vi "Teleop.vi"(10 "Match Info":T1={"Autonomous Elapsed Seconds"=0.0, "TeleOp Elapsed Seconds"=0.0, "Disabled Elapsed Seconds"=0.0, "Visited Autonomous"=FALSE, "Visited TeleOp"=FALSE, "Visited Disabled"=FALSE, "Autonomous Settings"={"Autonomous Style"=enum."Independent", "VI Refnum"=refnum}}, 11 "Call Context":T2) -> ()   [LabVIEW 2019]
doc: "This VI is called for each TeleOp packet received from the DS where the robot is not disabled. It is often used to read from the joysticks and update I/O or to update setpoints for timed control loops. It should complete and return within 20 milliseconds or it may miss DS packets."
uses:
  <vilib>/Rock Robotics/Network Tables/NT Read Boolean.vi
  Robot Global Data.vi
  <vilib>/Rock Robotics/WPI/Joystick/WPI_JoystickArcadeMapping.vi
  <vilib>/Rock Robotics/Network Tables/NT Read Number.vi
  <vilib>/Rock Robotics/Network Tables/NT Write Boolean Array.vi
  <vilib>/Rock Robotics/Network Tables/NT Write Numeric Array.vi
  <vilib>/Rock Robotics/WPI/ThirdParty/JAS_Junk/TrajLib/Trajectory_Library.lvlib
  <vilib>/Rock Robotics/WPI/DriverStation/WPI_DriverStationMatch Info.ctl
  <vilib>/Rock Robotics/WPI/DriverStation/WPI_DriverStationDerivedRobotMode.ctl
panel:
  out "Sample Slider 0":dbl(slide) scale=0.0..5.0
  out "Sample Boolean 1":bool
  out "Sample Boolean 0":bool
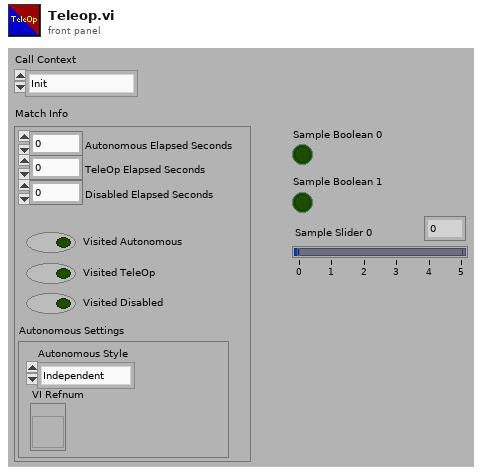
[diagram p1: front panel]
types:
  T1 = typedef "WPI_DriverStationMatch Info.ctl" = cluster{"Autonomous Elapsed Seconds":dbl, "TeleOp Elapsed Seconds":dbl, "Disabled Elapsed Seconds":dbl, "Visited Autonomous":bool, "Visited TeleOp":bool, "Visited Disabled":bool, "Autonomous Settings":cluster{"Autonomous Style":enum16{"Iterative", "Independent"}, "VI Refnum":refnum<vi>}}
  T2 = typedef "WPI_DriverStationDerivedRobotMode.ctl" = enum16{"Init", "Execute", "Stop"}
  T3 = typedef "WPI_JoystickDevRef.ctl" = cluster{"Device":T4}
  T4 = typedef "WPI_JoystickDeviceEnum.ctl" = enum16{"USB 0", "USB 1", "USB 2", "USB 3", "USB 4", "USB 5"}
  T5 = typedef "Trajectory_Library.lvlib/RAMSETE.ctl" = cluster{"B":dbl, "Zeta":dbl, "poseTolerance":T6, "poseError":T6, "Enabled":bool}
  T6 = typedef "Trajectory_Library.lvlib/POSE2D.ctl" = cluster{"TRANSLATION":T7, "ROTATION":T8}
  T7 = typedef "Trajectory_Library.lvlib/TRANSLATION2D.ctl" = cluster{"X":dbl, "Y":dbl}
  T8 = typedef "Trajectory_Library.lvlib/ROTATION2D.ctl" = cluster{"VALUE":dbl, "COS":dbl, "SIN":dbl}
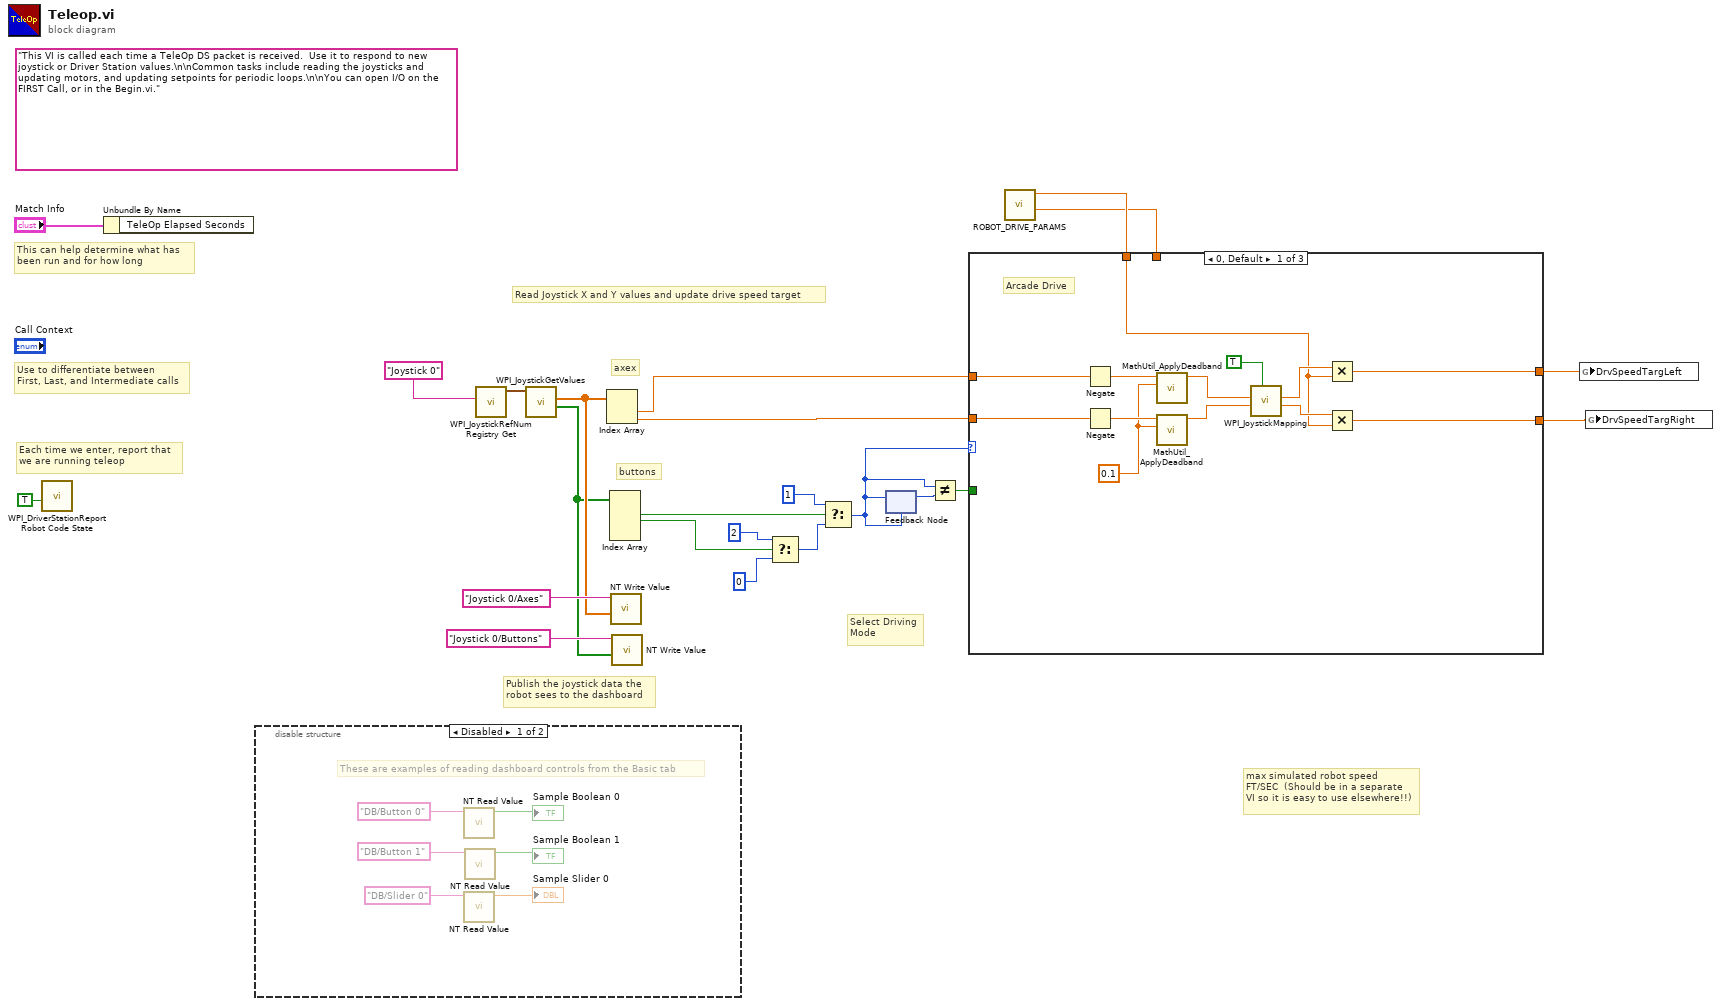
[diagram p0: block diagram]
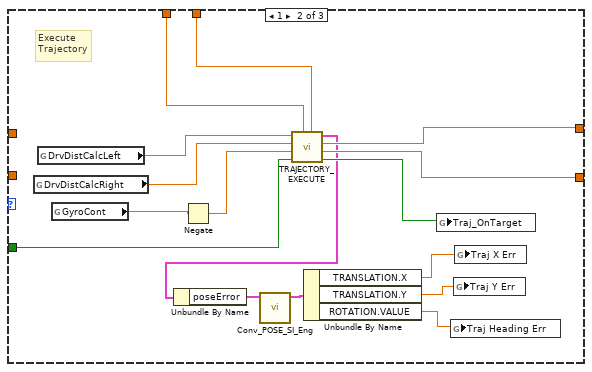
[diagram p2: hidden frame]
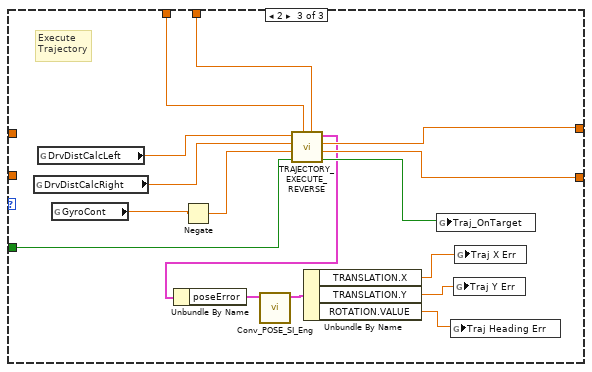
[diagram p3: hidden frame]
diagram:
  (unwired) "This VI is called each time a TeleOp DS packet is received.  Use it to respond to new joystick or Driver Station values.\n\nCommon tasks include reading the joysticks and updating motors, and updating setpoints for periodic loops.\n\nYou can open I/O on the FIRST Call, or in the Begin.vi."
  # "Select Driving\nMode"
  # "buttons"
  # "axex"
  # "max simulated robot speed\nFT/SEC  (Should be in a separate\nVI so it is easy to use elsewhere!!)"
  # "Publish the joystick data the\nrobot sees to the dashboard"
  # "Each time we enter, report that\nwe are running teleop"
  # "Use to differentiate between\nFirst, Last, and Intermediate calls"
  # "This can help determine what has\nbeen run and for how long"
  # "Read Joystick X and Y values and update drive speed target"
  n1 = call <vilib>:"WPI_DriverStationReport Robot Code State.vi"("TeleOp"=TRUE ("Autonomous")) -> ()  [unwired: 10 in, 1 out]
  n2 = Unbundle By Name("Match Info") -> ()  [unwired: 1 out]
  n3 = disable-structure shown="Disabled" {
    frame Disabled {
      # "These are examples of reading dashboard controls from the Basic tab"
      n4 = call-poly <vilib>:"NT Read Value.vi"("Name"="DB/Button 0" ("refnum name")) -> ("Boolean"=→"Sample Boolean 0":bool)  [unwired: 9 in, 1 out]
      n5 = call-poly <vilib>:"NT Read Value.vi"("Name"="DB/Slider 0" ("refnum name")) -> ("Numeric"=→"Sample Slider 0":dbl)  [unwired: 9 in, 1 out]
      n6 = call-poly <vilib>:"NT Read Value.vi"("Name"="DB/Button 1" ("refnum name")) -> ("Boolean"=→"Sample Boolean 1":bool)  [unwired: 9 in, 1 out]
    }
    frame Enabled {
    }
  }
  n7 = call <vilib>:"WPI_JoystickRefNum Registry Get.vi"("refnum name"="Joystick 0") -> ("JoystickDevRef"=w21:T3)  [unwired: 1 in, 9 out]
  n8 = call <vilib>:"WPI_JoystickGetValues.vi"("JoystickDevRef"=w21) -> ("Buttons"=w12:bool[], "Axes"=w17:dbl[])  [unwired: 6 in, 3 out]
  n9 = Index Array(array=w17) -> (element #1=w16:dbl, element #2=w15:dbl)  [unwired: 2 in]
  n10 = Index Array(array=w12) -> (element #1=w10:bool, element #2=w3:bool)  [unwired: 4 in, 2 out]
  n11 = call-poly <vilib>:"NT Write Value.vi"("Numeric Array"=w17, "Name"="Joystick 0/Axes") -> ()  [unwired: 9 in, 1 out]
  n12 = call-poly <vilib>:"NT Write Value.vi"("Boolean Array"=w12, "Name"="Joystick 0/Buttons") -> ()  [unwired: 9 in, 1 out]
  n13 = Select(t=2, s=w3, f=0) -> (s? t:f=w4:i32)
  n14 = Select(t=1, s=w10, f=w4) -> (s? t:f=w8:i32)
  n15 = feedback-in #1(w8) -> ()
  n16 = feedback #1(w8) -> (w9:i32)
  n17 = Not Equal?(x=w8, y=w9) -> (x != y?=w7:bool)
  n18 = call "ROBOT_DRIVE_PARAMS.vi"() -> ("Effective Wheelbase Ft"=w1:dbl, "Max Speed Ft/Sec"=w2:dbl)  [unwired: 10 in]
  n19 = case shown="0, Default" w8 {
    tunnel: w16 -> [w41 _ _]
    tunnel: w15 -> [w40 _ _]
    tunnel: [w39 w52 w68] -> w14
    tunnel: [w38 w51 w67] -> w13
    tunnel: w2 -> [w35 w53 w69]
    tunnel: w7 -> [_ w58 w74]
    tunnel: w1 -> [_ w43 w59]
    frame 0, Default {
      w30 = 0.1 ("Deadband")
      # "Arcade Drive"
      n20 = Negate(x=w41) -> (-x=w34:dbl)
      n21 = Negate(x=w40) -> (-x=w32:dbl)
      n22 = call <vilib>:"MathUtil_ApplyDeadband.vi"("Deadband"=w30, "Value"=w34) -> ("Result"=w33:dbl)  [unwired: 9 in]
      n23 = call <vilib>:"MathUtil_ApplyDeadband.vi"("Deadband"=w30, "Value"=w32) -> ("Result"=w31:dbl)  [unwired: 9 in]
      n24 = call-poly <vilib>:"WPI_JoystickMapping.vi"("Square Inputs"=TRUE, "Y axis value"=w31, "X axis value"=w33) -> ("Right Motor Value"=w36:dbl, "Left Motor Value"=w37:dbl)  [unwired: 7 in]
      n25 = Multiply(x=w37, y=w35) -> (x*y=w39:dbl)
      n26 = Multiply(x=w36, y=w35) -> (x*y=w38:dbl)
    }
    frame 1 {
      # "Execute\nTrajectory"
      n27 = global read "Robot Global Data.vi" "DrvDistCalcRight"() -> (w55:dbl)
      n28 = global read "Robot Global Data.vi" "DrvDistCalcLeft"() -> (w56:dbl)
      n29 = global read "Robot Global Data.vi" "GyroCont"() -> (w57:dbl)
      n30 = Negate(x=w57) -> (-x=w54:dbl)
      n31 = call "TRAJECTORY_EXECUTE.vi"("Track Width FT"=w43, "Max Speed\nFT/SEC"=w53, "Init"=w58, "Gyro Continous\n (inc counterclockwise)"=w54, "Right Distance"=w55, "Left Distance"=w56) -> ("AtReference"=w50:bool, "Right Speed Target"=w51:dbl, "Left Speed Target"=w52:dbl, "outRAMSETE (SI)"=w49:T5)  [unwired: 1 in, 1 out]
      n32 = Unbundle By Name(w49) -> ("poseError"=w48:T6)
      n33 = call <vilib>:"Conv_POSE_SI_Eng.vi"("Err Pose in SI"=w48) -> ("Err Pose out ENG"=w47:T6)  [unwired: 10 in]
      n34 = Unbundle By Name(w47) -> ("TRANSLATION.X"=w46:dbl, "TRANSLATION.Y"=w45:dbl, "ROTATION.VALUE"=w44:dbl)
      n35 = global write "Robot Global Data.vi" "Traj_OnTarget"(w50) -> ()
      n36 = global write "Robot Global Data.vi" "Traj Heading Err"(w44) -> ()
      n37 = global write "Robot Global Data.vi" "Traj Y Err"(w45) -> ()
      n38 = global write "Robot Global Data.vi" "Traj X Err"(w46) -> ()
    }
    frame 2 {
      # "Execute\nTrajectory"
      n39 = global read "Robot Global Data.vi" "DrvDistCalcRight"() -> (w71:dbl)
      n40 = global read "Robot Global Data.vi" "DrvDistCalcLeft"() -> (w72:dbl)
      n41 = global read "Robot Global Data.vi" "GyroCont"() -> (w73:dbl)
      n42 = Negate(x=w73) -> (-x=w70:dbl)
      n43 = call "TRAJECTORY_EXECUTE_REVERSE.vi"("Track Width FT"=w59, "Max Speed\nFT/SEC"=w69, "Init"=w74, "Gyro Continous\n (inc counterclockwise)"=w70, "Right Distance"=w71, "Left Distance"=w72) -> ("AtReference"=w66:bool, "Right Speed Target"=w67:dbl, "Left Speed Target"=w68:dbl, "outRAMSETE (SI)"=w65:T5)  [unwired: 1 in, 1 out]
      n44 = Unbundle By Name(w65) -> ("poseError"=w64:T6)
      n45 = call <vilib>:"Conv_POSE_SI_Eng.vi"("Err Pose in SI"=w64) -> ("Err Pose out ENG"=w63:T6)  [unwired: 10 in]
      n46 = Unbundle By Name(w63) -> ("TRANSLATION.X"=w62:dbl, "TRANSLATION.Y"=w61:dbl, "ROTATION.VALUE"=w60:dbl)
      n47 = global write "Robot Global Data.vi" "Traj_OnTarget"(w66) -> ()
      n48 = global write "Robot Global Data.vi" "Traj Heading Err"(w60) -> ()
      n49 = global write "Robot Global Data.vi" "Traj Y Err"(w61) -> ()
      n50 = global write "Robot Global Data.vi" "Traj X Err"(w62) -> ()
    }
  }
  n51 = global write "Robot Global Data.vi" "DrvSpeedTargLeft"(w14) -> ()
  n52 = global write "Robot Global Data.vi" "DrvSpeedTargRight"(w13) -> ()
